vi "SMTP Email Extract Address.vi"(7 "string with address":string) -> (1 "error":bool, 2 "string after address":string, 3 "address":string)   [LabVIEW 2011, in "NewNI_SMTPEmail.lvlib"]
doc: "Extracts the first valid email address from a string."
uses:
  NewNI_SMTPEmail.lvlib
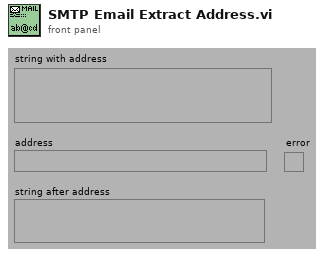
[diagram p1: front panel]
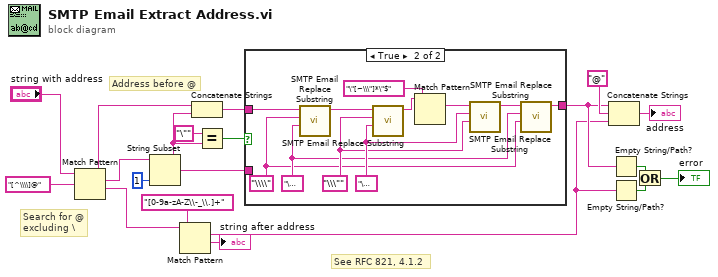
[diagram p0: block diagram]
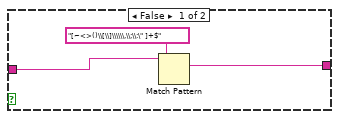
[diagram p2: hidden frame]
diagram:
  # "Address before @"
  # "Search for @\nexcluding \\"
  # "See RFC 821, 4.1.2"
  n1 = Match Pattern(string="string with address", regular expression="[^\\\\]@") -> (before substring=w13:string, match substring=w18:string, after substring=w8:string)  [unwired: 2 out]
  n2 = String Subset(string=w18, length (rest)=1 ("length")) -> (substring=w16:string)  [unwired: 1 out]
  n3 = Match Pattern(string=w8, regular expression="[0-9a-zA-Z\\-_\\.]+") -> (match substring=w5:string, after substring=→"string after address":string)  [unwired: 3 out]
  n4 = Concatenate Strings(w13, w16) -> (w12:string)
  n5 = Equal?(x="\"", y=w16) -> (x = y?=w14:bool)
  n6 = case shown="True" w14 {
    tunnel: w16 -> [_ _]
    tunnel: w12 -> [w21 w32]
    tunnel: [w20 w23] -> w6
    frame False {
      n7 = Match Pattern(string=w21, regular expression="[~<>()\\[\\]\\\\\\,\\;\\:\" ]+$") -> (match substring=w20:string)  [unwired: 4 out]
    }
    frame True {
      w26 = "\\\"" ("delimiter ([\\s\\t\\n\\r]+)")
      w27 = "\u0001" ("delimiter ([\\s\\t\\n\\r]+)")
      w25 = "\u0000" ("delimiter ([\\s\\t\\n\\r]+)")
      w24 = "\\\\" ("delimiter ([\\s\\t\\n\\r]+)")
      n8 = call "SMTP Email Replace Substring.vi"("replacement"=w25, "pattern"=w24, "text"=w32) -> ("text out"=w31:string)  [unwired: 4 in, 4 out]
      n9 = call "SMTP Email Replace Substring.vi"("replacement"=w27, "pattern"=w26, "text"=w31) -> ("text out"=w30:string)  [unwired: 4 in, 4 out]
      n10 = Match Pattern(string=w30, regular expression="\"[~\\\"]*\"$") -> (match substring=w28:string)  [unwired: 4 out]
      n11 = call "SMTP Email Replace Substring.vi"("replacement"=w26, "pattern"=w27, "text"=w28) -> ("text out"=w29:string)  [unwired: 4 in, 4 out]
      n12 = call "SMTP Email Replace Substring.vi"("replacement"=w24, "pattern"=w25, "text"=w29) -> ("text out"=w23:string)  [unwired: 4 in, 4 out]
    }
  }
  n13 = Concatenate Strings(w6, "@" ("delimiter ([\\s\\t\\n\\r]+)"), w5) -> (→"address":string)
  n14 = Empty String/Path?(string/path=w6) -> (empty?=w4:bool)
  n15 = Empty String/Path?(string/path=w5) -> (empty?=w3:bool)
  n16 = Or(x=w4, y=w3) -> (x .or. y?=→"error":bool)
